vi "niFPGA BFGroup Twiddle Table 128 U64 Inv.vi"(7 "address":fxp<+,7,7>) -> (4 "twid real":fxp<+/-,33,2> format="%.32g", 6 "twid imag":fxp<+/-,33,2> format="%.32g")   [LabVIEW 2017]
uses:
  <vilib>/rvi/FXPMathLib/basic elements/FxpDiscreteDelay/XNode/nifxpmath_DiscreteDelay.xnode
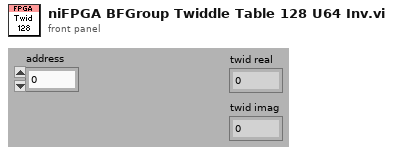
[diagram p1: front panel]
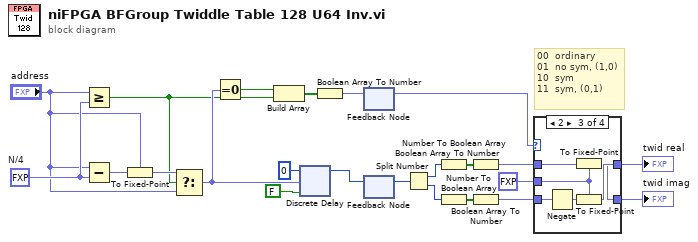
[diagram p0: block diagram]
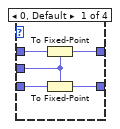
[diagram p2: hidden frame]
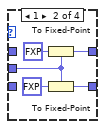
[diagram p3: hidden frame]
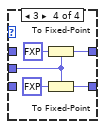
[diagram p4: hidden frame]
diagram:
  w18 = fxp<+,7,7> 64.0  # N/4
  # "00  ordinary\n01  no sym, (1,0)\n10  sym\n11  sym, (0,1)"
  n1 = Greater Or Equal?(x="address", y=w18) -> (x >= y?=w6:bool)
  n2 = Subtract(x="address", y=w18) -> (x-y=w17:fxp<+/-,8,8>)
  n3 = To Fixed-Point(fixed-point type="address", number=w17) -> (fixed-point=w16:fxp<+,7,7>)
  n4 = Select(t=w16, s=w6, f="address") -> (s? t:f=w10:fxp<+,7,7>)
  n5 = Equal To 0?(x=w10) -> (x = 0?=w7:bool)
  n6 = Build Array(w7, w6) -> (w8:bool[])
  n7 = xnode "Discrete Delay"("D"=u64 0, "n-1[0..63]"=w10, "enable"=FALSE) -> ("Q"=w9:u64)
  n8 = Boolean Array To Number(Boolean array=w8) -> (number=w5:fxp<+,2,2>)
  n9 = feedback-in #1(w5) -> ()
  n10 = feedback #1() -> (w4:fxp<+,2,2>)  [unwired: 1 out]
  n11 = feedback-in #2(w9) -> ()
  n12 = feedback #2() -> (w19:u64)  [unwired: 1 out]
  n13 = Split Number(x=w19) -> (hi(x)=w22:u32, lo(x)=w20:u32)
  n14 = Number To Boolean Array(number=w22) -> (Boolean array=w23:bool[])
  n15 = Number To Boolean Array(number=w20) -> (Boolean array=w21:bool[])
  n16 = Boolean Array To Number(Boolean array=w23) -> (number=w14:fxp<+/-,32,1>)
  n17 = Boolean Array To Number(Boolean array=w21) -> (number=w13:fxp<+/-,32,1>)
  n18 = case shown="2" w4 {
    tunnel: w14 -> [w28 _ w36 _]
    tunnel: [w27 w32 w37 w43] -> w2
    tunnel: w13 -> [w26 _ w38 _]
    tunnel: [w25 w30 w34 w41] -> w1
    tunnel: fxp<+/-,33,2> 0.0 ("fixed-point type") -> [w24 w29 w35 w40]
    frame 0, Default {
      n19 = To Fixed-Point(fixed-point type=w24, number=w28) -> (fixed-point=w27:fxp<+/-,33,2>)
      n20 = To Fixed-Point(fixed-point type=w24, number=w26) -> (fixed-point=w25:fxp<+/-,33,2>)
    }
    frame 1 {
      n21 = To Fixed-Point(fixed-point type=w29, number=fxp<+,1,1> 1.0 ("fixed-point type")) -> (fixed-point=w32:fxp<+/-,33,2>)
      n22 = To Fixed-Point(fixed-point type=w29, number=fxp<+,1,1> 0.0 ("fixed-point type")) -> (fixed-point=w30:fxp<+/-,33,2>)
    }
    frame 2 {
      n23 = Negate(x=w38) -> (-x=w39:fxp<+/-,33,2>)
      n24 = To Fixed-Point(fixed-point type=w35, number=w36) -> (fixed-point=w34:fxp<+/-,33,2>)
      n25 = To Fixed-Point(fixed-point type=w35, number=w39) -> (fixed-point=w37:fxp<+/-,33,2>)
    }
    frame 3 {
      n26 = To Fixed-Point(fixed-point type=w40, number=fxp<+,1,1> 0.0 ("fixed-point type")) -> (fixed-point=w43:fxp<+/-,33,2>)
      n27 = To Fixed-Point(fixed-point type=w40, number=fxp<+,1,1> 1.0 ("fixed-point type")) -> (fixed-point=w41:fxp<+/-,33,2>)
    }
  }
  "twid real" <- w2
  "twid imag" <- w1
